vi "settings.vi"(3 "error in (no error)":errorcluster, 4 "values":dbl[](array[numeric]), 5 "sturing in":refnum<visa-resource-name>) -> (0 "error out":errorcluster, 1 "String":string, 2 "sturing out":refnum<visa-resource-name>)   [LabVIEW 2019]
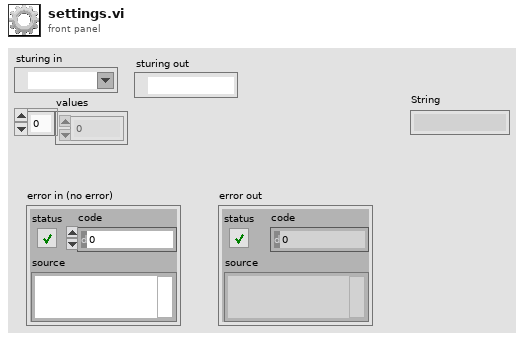
[diagram p1: front panel]
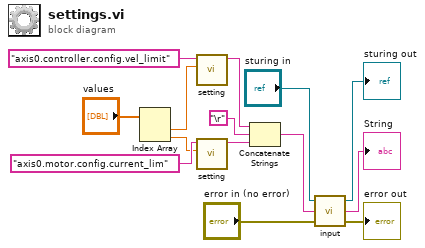
[diagram p0: block diagram]
diagram:
  n1 = Index Array(array="values") -> (element #1=w13:dbl, element #2=w10:dbl)  [unwired: 2 in]
  n2 = call "setting.vi"("value"=w13, "setting"="axis0.controller.config.vel_limit") -> ("write"=w12:string)  [unwired: 9 in]
  n3 = call "setting.vi"("value"=w10, "setting"="axis0.motor.config.current_lim") -> ("write"=w8:string)  [unwired: 9 in]
  n4 = Concatenate Strings(w12, "\r", w8) -> (w6:string)
  n5 = call "input.vi"("error in (no error)"="error in (no error)", "commando"=w6, "VISA in"="sturing in") -> ("error out"=→"error out":errorcluster, "DEBUG"=→"String":string, "VISA out"=→"sturing out":refnum<visa-resource-name>)
